vi "ArmExecute.vi"   [LabVIEW 2023]
doc: "Execute Arm VI's\nInputs:\n\nOutputs:"
uses:
  ArmGamePiecePreset.ctl
  <vilib>/Rock Robotics/WPI/ThirdParty/JAS_Junk/TrajLib/Timer_New.vi
  <vilib>/Utility/semaphor.llb/Obtain Semaphore Reference.vi
  <vilib>/Rock Robotics/WPI/ThirdParty/JAS_Junk/TrajLib/Timer_Reset.vi
  <vilib>/Rock Robotics/WPI/ThirdParty/JAS_Junk/TrajLib/Timer_Start.vi
  <vilib>/Rock Robotics/WPI/ThirdParty/JAS_Junk/TrajLib/Timer_HasPeriodPassedOnce.vi
  ArmGlobal.vi
  <vilib>/Rock Robotics/Network Tables/NT Write Boolean.vi
  <vilib>/Rock Robotics/WPI/ThirdParty/JAS_Junk/TrajLib/Trajectory_Library.lvlib
  <vilib>/Rock Robotics/WPI/ThirdParty/PhotonVisionLib/PhotonVisionLib.lvlib
types:
  T1 = typedef "ArmGamePiecePreset.ctl" = enum16{"Cube", "Cone"}
  T2 = typedef "WPI_MotorControlDeviceRef.ctl" = cluster{"DeviceStatus":errorcluster, "Type":T3, "PWM":cluster{"PWM Channel":T4, "DeadBand":T5}, "CAN":cluster{"Device Number":u8, "SetOutput VI Ref":variant, "GetOutput VI Ref":variant, "Enable VI Ref":variant, "Disable VI Ref":variant, "Data":variant}, "Invert":bool, "DIO PWM":cluster{"PWM \"Enable\" Channel":T4, "DIOChannel":T6, "PWM Rate":dbl}}
  T3 = typedef "WPI_MotorControlType.ctl" = enum16{"PWM", "CAN", "DIO PWM"}
  T4 = typedef "FPGA_DIOPWMChannel.ctl" = enum8{"PWM 0", "PWM 1", "PWM 2", "PWM 3", "PWM 4", "PWM 5", "PWM 6", "PWM 7", "PWM 8", "PWM 9", "PWM MXP 0", "PWM MXP 1", "PWM MXP 2", "PWM MXP 3", "PWM MXP 4", "PWM MXP 5", "PWM MXP 6", "PWM MXP 7", "PWM MXP 8", "PWM MXP 9", "Invalid"}
  T5 = typedef "WPI_PWMDeadband.ctl" = cluster{"Name":string, "maxPositivePwm":i32, "minPositivePwm":i32, "centerPwm":i32, "maxNegativePwm":i32, "minNegativePwm":i32, "angularRange":u16}
  T6 = typedef "FPGA_DIOChannel.ctl" = enum8{"DIO 0", "DIO 1", "DIO 2", "DIO 3", "DIO 4", "DIO 5", "DIO 6", "DIO 7", "DIO 8", "DIO 9", "DIO MXP 0", "DIO MXP 1", "DIO MXP 2", "DIO MXP 3", "DIO MXP 4", "DIO MXP 5", "DIO MXP 6", "DIO MXP 7", "DIO MXP 8", "DIO MXP 9", "DIO MXP 10", "DIO MXP 11", "DIO MXP 12", "DIO MXP 13", "DIO MXP 14", "DIO MXP 15", "SPI Port CS1", "SPI Port CS2", "SPI Port CS3", "SPI Port MISO", "SPI Port MOSI", "Invalid"}
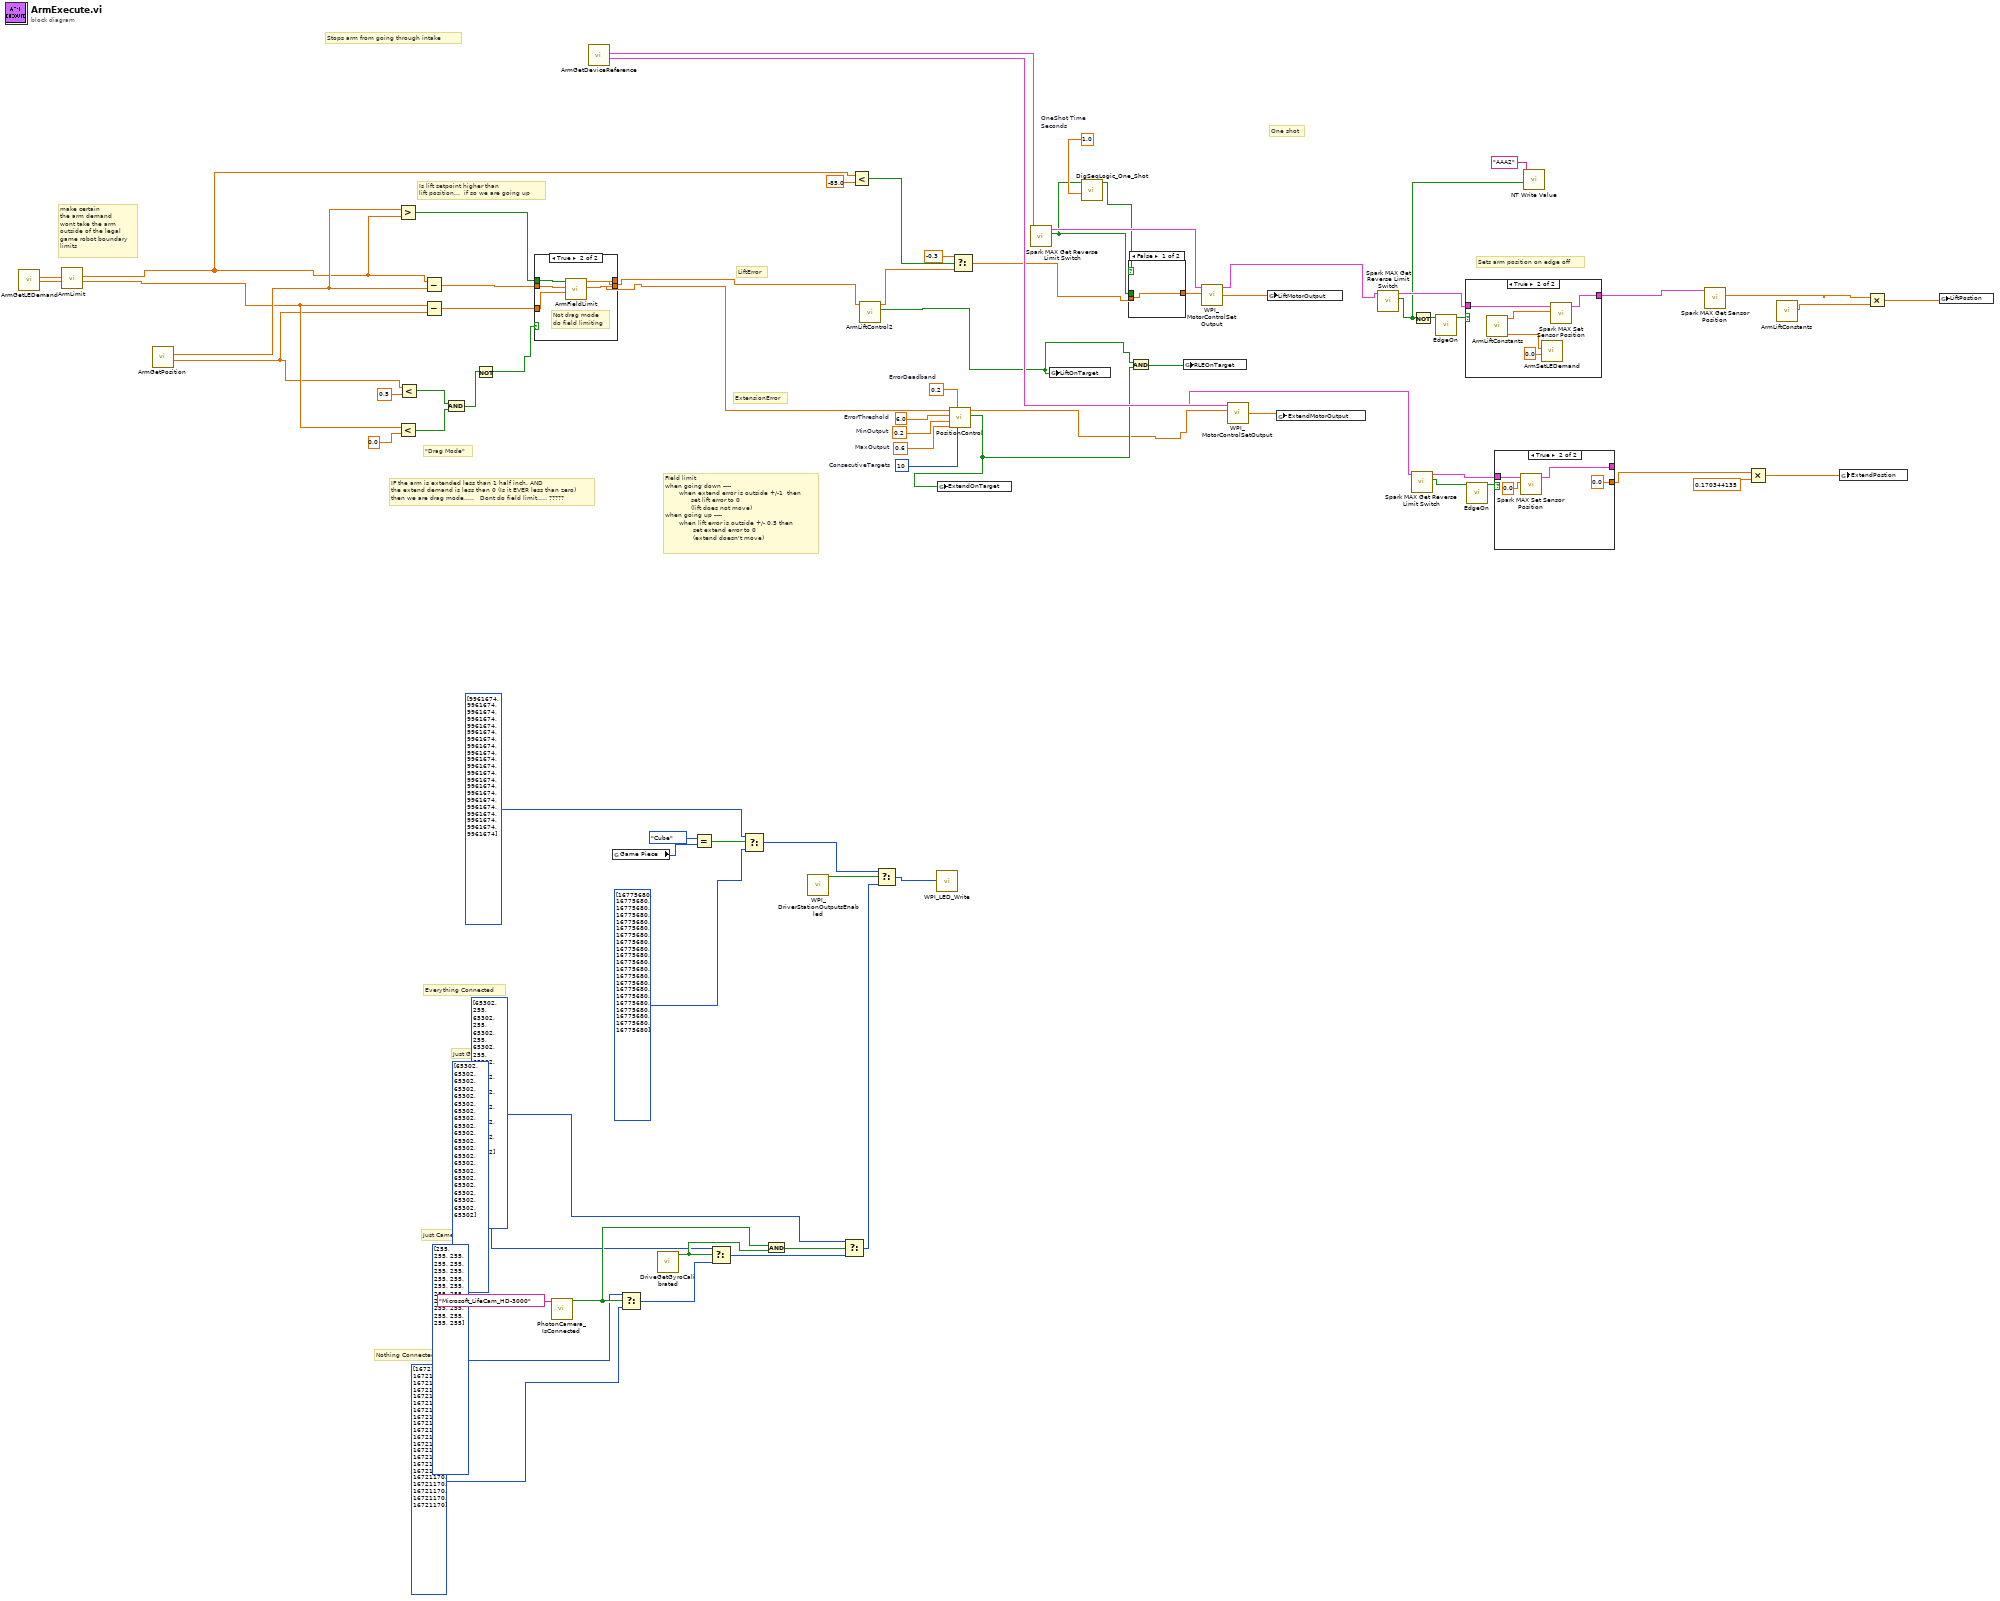
[diagram p0: block diagram]
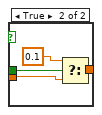
[diagram p2: hidden frame]
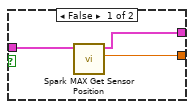
[diagram p5: hidden frame]
diagram:
  w23 = 1.0  # OneShot Time Seconds
  w69 = 10  # ConsecutiveTargets
  w70 = 0.6  # MaxOutput
  w71 = 0.2  # MinOutput
  w72 = 6.0  # ErrorThreshold
  w73 = 0.2  # ErrorDeadband
  # "make certain\nthe arm demand\nwont take the arm\noutside of the legal\ngame robot boundary\nlimits"
  # "FIeld limit\nwhen going down ----\n       when extend error is outside +/-1  then\n             set lift error to 0\n             (lift does not move)\nwhen going up ----\n       when lift error is outside +/- 0.5 then\n              set extend error to 0\n              (extend doesn't move)"
  # "IF the arm is extended less than 1 half inch. AND\nthe extend demand is less than 0 (Is it EVER less than zero)\nthen we are drag mode.....   Dont do field limit..... ?????"
  # "Is lift setpoint higher than\nlift position...  if so we are going up"
  # "Everything Connected"
  # "Just Gyro"
  # "Just Camera"
  # "Nothing Connected"
  # "One shot"
  # "Sets arm position on edge off"
  # "\"Drag Mode\""
  # "Stops arm from going through intake"
  # "ExtensionError"
  # "LiftError"
  n1 = call "ArmGetLEDemand.vi"() -> ("ExtendPositonDemand(in)"=w61:dbl, "LiftPositionDemand(d)"=w62:dbl)  [unwired: 10 in]
  n2 = call "ArmLimit.vi"("Extend"=w61, "Lift"=w62) -> ("Extend"=w29:dbl, "Lift"=w37:dbl)  [unwired: 8 in]
  n3 = call "ArmGetPosition.vi"() -> ("ExtendPostion"=w26:dbl, "LiftPostion"=w50:dbl)  [unwired: 10 in]
  n4 = Greater?(x=w50, y=w37) -> (0:w53:bool)
  n5 = Less?(x=w29, y=0.0) -> (x < y?=w27:bool)
  n6 = Less?(x=w26, y=0.5) -> (x < y?=w28:bool)
  n7 = Subtract(x=w37, y=w50) -> (x-y=w49:dbl)
  n8 = Subtract(x=w29, y=w26) -> (x-y=w54:dbl)
  n9 = And(x=w28, y=w27) -> (x .and. y?=w24:bool)
  n10 = Not(x=w24) -> (.not. x?=w20:bool)
  n11 = case shown="True" w20 {
    tunnel: w54 -> [w77 w83]
    tunnel: w49 -> [w78 w82]
    tunnel: w53 -> [_ w81]
    tunnel: [w78 w80] -> w52
    tunnel: [w77 w79] -> w51
    frame False {
    }
    frame True {
      # "Not drag mode\ndo field limiting"
      n12 = call "ArmFieldLimit.vi"("Extend Error"=w83, "Lift Error"=w82, "Going Down?"=w81) -> ("Extend Error"=w79:dbl, "Lift Error"=w80:dbl)  [unwired: 7 in]
    }
  }
  n13 = call <vilib>:"PhotonCamera_IsConnected.vi"("CameraName"="Microsoft_LifeCam_HD-3000") -> ("IsConnected"=w4:bool)  [unwired: 9 in, 1 out]
  n14 = call "ArmGetDeviceReference.vi"() -> ("armExtend"=w76:T2, "armLift"=w41:T2)  [unwired: 10 in]
  n15 = global read "ArmGlobal.vi" "Game Piece"() -> (w19:T1)
  n16 = Select(t=u32[] [255, 255, 255, 255, 255, 255, 255, 255, 255, 255, 255, 255, 255, 255, 255, 255, 255, 255, 255, 255, 255] ("Color Array"), s=w4, f=u32[] [16721170, 16721170, 16721170, 16721170, 16721170, 16721170, 16721170, 16721170, 16721170, 16721170, 16721170, 16721170, 16721170, 16721170, 16721170, 16721170, 16721170, 16721170, 16721170, 16721170, 16721170] ("Color Array")) -> (s? t:f=w9:u32[])
  n17 = call "DriveGetGyroCalibrated.vi"() -> ("GryoCalibrated"=w5:bool)  [unwired: 11 in]
  n18 = Equal?(x=ArmGamePiecePreset."Cube", y=w19) -> (x = y?=w17:bool)
  n19 = Select(t=u32[] [65302, 65302, 65302, 65302, 65302, 65302, 65302, 65302, 65302, 65302, 65302, 65302, 65302, 65302, 65302, 65302, 65302, 65302, 65302, 65302, 65302] ("Color Array"), s=w5, f=w9) -> (s? t:f=w7:u32[])
  n20 = Select(t=u32[] [9961674, 9961674, 9961674, 9961674, 9961674, 9961674, 9961674, 9961674, 9961674, 9961674, 9961674, 9961674, 9961674, 9961674, 9961674, 9961674, 9961674, 9961674, 9961674, 9961674, 9961674] ("Color Array"), s=w17, f=u32[] [16775680, 16775680, 16775680, 16775680, 16775680, 16775680, 16775680, 16775680, 16775680, 16775680, 16775680, 16775680, 16775680, 16775680, 16775680, 16775680, 16775680, 16775680, 16775680, 16775680, 16775680] ("Color Array")) -> (s? t:f=w13:u32[])
  n21 = And(x=w4, y=w5) -> (x .and. y?=w6:bool)
  n22 = call <vilib>:"WPI_DriverStationOutputsEnabled.vi"() -> ("OutputsEnabled?"=w12:bool)  [unwired: 10 in, 1 out]
  n23 = Select(t=u32[] [65302, 255, 65302, 255, 65302, 255, 65302, 255, 65302, 255, 65302, 255, 65302, 255, 65302, 255, 65302, 255, 65302, 255, 65302] ("Color Array"), s=w6, f=w7) -> (s? t:f=w11:u32[])
  n24 = Less?(x=w37, y=-85.0) -> (x < y?=w36:bool)
  n25 = call "ArmLiftControl2.vi"("erronIn(d)"=w52) -> ("OnTarget"=w55:bool, "motorOutput"=w34:dbl)  [unwired: 9 in]
  n26 = Select(t=w13, s=w12, f=w11) -> (s? t:f=w14:u32[])
  n27 = call <vilib>:"WPI_LED_Write.vi"("Color Array"=w14) -> ()  [unwired: 10 in, 1 out]
  n28 = call "PositionControl.vi"("ConsecutiveTargets"=w69, "ErrorDeadband"=w73, "MaxOutput"=w70, "MinOutput"=w71, "ErrorThreshold"=w72, "Error"=w51) -> ("OnTarget"=w68:bool, "OutputValue"=w44:dbl)  [unwired: 3 in, 1 out]
  n29 = global write "ArmGlobal.vi" "ExtendOnTarget"(w68) -> ()
  n30 = Select(t=-0.3, s=w36, f=w34) -> (s? t:f=w35:dbl)
  n31 = call <vilib>:"Spark MAX Get Reverse Limit Switch.vi"("MotorControlDevRef in"=w41) -> ("Hard Limit Rev"=w22:bool, "MotorControlDevRef out"=w42:T2)  [unwired: 7 in, 2 out]
  n32 = global write "ArmGlobal.vi" "LiftOnTarget"(w55) -> ()
  n33 = call <vilib>:"DigSeqLogic_One_Shot.vi"("OneShot"=w23, "Input"=w22) -> ("Output"=w21:bool)  [unwired: 8 in, 1 out]
  n34 = case shown="False" w21 {
    tunnel: [w84 w88] -> w57
    tunnel: w35 -> [w84 w86]
    tunnel: w22 -> [_ w85]
    frame False {
    }
    frame True {
      n35 = Select(t=0.1, s=w85, f=w86) -> (s? t:f=w88:dbl)
    }
  }
  n36 = And(x=w55, y=w68) -> (x .and. y?=w67:bool)
  n37 = global write "ArmGlobal.vi" "RLEOnTarget"(w67) -> ()
  n38 = call <vilib>:"WPI_MotorControlSetOutput.vi"("Output"=w57, "MotorControlDevRef"=w42) -> ("Motor Output"=w74:dbl, "MotorControlDevRef"=w43:T2)  [unwired: 7 in, 1 out]
  n39 = call <vilib>:"WPI_MotorControlSetOutput.vi"("Output"=w44, "MotorControlDevRef"=w76) -> ("Motor Output"=w75:dbl, "MotorControlDevRef"=w63:T2)  [unwired: 7 in, 1 out]
  n40 = global write "ArmGlobal.vi" "LiftMotorOutput"(w74) -> ()
  n41 = global write "ArmGlobal.vi" "ExtendMotorOutput"(w75) -> ()
  n42 = call <vilib>:"Spark MAX Get Reverse Limit Switch.vi"("MotorControlDevRef in"=w43) -> ("Hard Limit Rev"=w39:bool, "MotorControlDevRef out"=w47:T2)  [unwired: 7 in, 2 out]
  n43 = call <vilib>:"Spark MAX Get Reverse Limit Switch.vi"("MotorControlDevRef in"=w63) -> ("Hard Limit Rev"=w32:bool, "MotorControlDevRef out"=w59:T2)  [unwired: 7 in, 2 out]
  n44 = Not(x=w39) -> (.not. x?=w45:bool)
  n45 = call "EdgeOn.vi"("Current State"=w45) -> ("Edge On Found"=w46:bool)  [unwired: 10 in]
  n46 = case shown="True" w46 {
    tunnel: w47 -> [w89 w94]
    tunnel: [w89 w93] -> w48
    frame False {
    }
    frame True {
      n47 = call "ArmLiftConstants.vi"() -> ("Starting Angle"=w90:dbl, "StartingArmPos"=w92:dbl)  [unwired: 8 in, 2 out]
      n48 = call "ArmSetLEDemand.vi"("SetExtendPositonDemand(in)"=0.0, "SetLIftPostionDemand(d)"=w90) -> ()  [unwired: 10 in]
      n49 = call <vilib>:"Spark MAX Set Sensor Position.vi"("Position"=w92, "MotorControlDeviceRef"=w94) -> ("MotorControlDeviceRef"=w93:T2)  [unwired: 8 in, 1 out]
    }
  }
  n50 = call "EdgeOn.vi"("Current State"=w32) -> ("Edge On Found"=w58:bool)  [unwired: 10 in]
  n51 = case shown="True" w58 {
    tunnel: w59 -> [w97 w101]
    tunnel: [w96 w100] -> _
    tunnel: [w95 0.0 ("Sensor Position")] -> w31
    frame False {
      n52 = call <vilib>:"Spark MAX Get Sensor Position.vi"("MotorControlDevRef in"=w97) -> ("Sensor Position"=w95:dbl, "MotorControlDevRef out"=w96:T2)  [unwired: 7 in, 2 out]
    }
    frame True {
      n53 = call <vilib>:"Spark MAX Set Sensor Position.vi"("Position"=0.0, "MotorControlDeviceRef"=w101) -> ("MotorControlDeviceRef"=w100:T2)  [unwired: 8 in, 1 out]
    }
  }
  n54 = call-poly <vilib>:"NT Write Value.vi"("value"=w39, "name"="AAA2") -> ()  [unwired: 9 in, 1 out]
  n55 = call <vilib>:"Spark MAX Get Sensor Position.vi"("MotorControlDevRef in"=w48) -> ("Sensor Position"=w64:dbl)  [unwired: 7 in, 3 out]
  n56 = Multiply(x=w31, y=0.170344135) -> (x*y=w60:dbl)
  n57 = call "ArmLiftConstants.vi"() -> ("LiftConversionFactor"=w56:dbl)  [unwired: 8 in, 3 out]
  n58 = global write "ArmGlobal.vi" "ExtendPostion"(w60) -> ()
  n59 = Multiply(x=w64, y=w56) -> (x*y=w66:dbl)
  n60 = global write "ArmGlobal.vi" "LiftPostion"(w66) -> ()
